vi "Get File Path.vi"(8 "error in (no error)":errorcluster, 11 "DSF Configuration Reference in":T1) -> (0 "error out":errorcluster, 2 "file path":path, 3 "DSF Configuration Reference out":T1, 5 "need update":bool)   [LabVIEW 2017, in "DSF Configuration API.lvlib"]
uses:
  DSF Configuration API.lvlib
  Controls/Session/DSF Configuration Reference.ctl
  Controls/DSF File Format/Internal.DSF Configuration.ctl
  Public/Controls/DSF Version Info.ctl
  Controls/DSF File Format/Internal.DSF Plugin with ID.ctl
  Controls/DSF File Format/Internal.DSF Plugin Info.ctl
  Public/Controls/DSF Timing Info.ctl
  Controls/DSF File Format/Internal.DSF Group with ID.ctl
  Controls/DSF File Format/Internal.DSF Group Info.ctl
  Controls/DSF File Format/Internal.DSF Transfer with ID.ctl
  Controls/DSF File Format/Internal.DSF Transfer Info.ctl
  Controls/DSF File Format/Internal.DSF Channel with ID.ctl
  Controls/DSF File Format/Internal.DSF Channel Info.ctl
  Controls/DSF File Format/Internal.DSF Settings with ID.ctl
  Controls/DSF File Format/Internal.DSF Settings Info.ctl
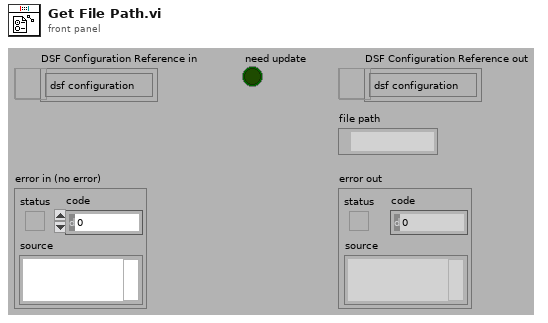
[diagram p1: front panel]
types:
  T1 = typedef "DSF Configuration API.lvlib/DSF Configuration Reference.ctl" = refnum<data-value>
  T2 = typedef "DSF Configuration API.lvlib/Internal.DSF Configuration.ctl" = cluster{"dsfversion":T3, "version":T3, "plugins":T4[], "groups":T7[], "transfers":T9[], "channels":T11[], "settings":T13[]}
  T3 = typedef "DSF Configuration API.lvlib/DSF Version Info.ctl" = cluster{"major":u32, "minor":u32, "fix":u32, "build":string}
  T4 = typedef "DSF Configuration API.lvlib/Internal.DSF Plugin with ID.ctl" = cluster{"id":string, "values":T5}
  T5 = typedef "DSF Configuration API.lvlib/Internal.DSF Plugin Info.ctl" = cluster{"type":string, "timing":T6, "group ids":string[], "settings id":string}
  T6 = typedef "DSF Configuration API.lvlib/DSF Timing Info.ctl" = cluster{"priority":u64, "decimation":u64, "offset":u64}
  T7 = typedef "DSF Configuration API.lvlib/Internal.DSF Group with ID.ctl" = cluster{"id":string, "values":T8}
  T8 = typedef "DSF Configuration API.lvlib/Internal.DSF Group Info.ctl" = cluster{"direction":i32, "timing":T6, "transfer ids":string[], "settings id":string}
  T9 = typedef "DSF Configuration API.lvlib/Internal.DSF Transfer with ID.ctl" = cluster{"id":string, "values":T10}
  T10 = typedef "DSF Configuration API.lvlib/Internal.DSF Transfer Info.ctl" = cluster{"byte order":i32, "channel ids":string[], "settings id":string}
  T11 = typedef "DSF Configuration API.lvlib/Internal.DSF Channel with ID.ctl" = cluster{"id":string, "values":T12}
  T12 = typedef "DSF Configuration API.lvlib/Internal.DSF Channel Info.ctl" = cluster{"count":u64, "buffer offset":u64, "data type":i32, "settings id":string}
  T13 = typedef "DSF Configuration API.lvlib/Internal.DSF Settings with ID.ctl" = cluster{"id":string, "values":T14}
  T14 = typedef "DSF Configuration API.lvlib/Internal.DSF Settings Info.ctl" = cluster{"key":string, "value":string}[]
  T15 = cluster{"dsf configuration":T2, "path":path, "dirty":bool}
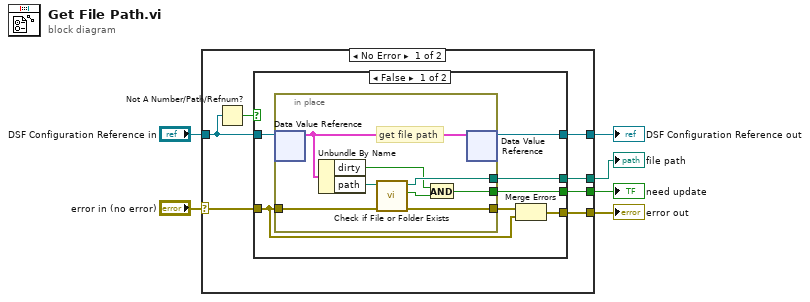
[diagram p0: block diagram]
diagram:
  n1 = case shown="No Error" "error in (no error)" {
    selector: "error in (no error)" -> [w10 w31]
    tunnel: "DSF Configuration Reference in" -> [w8 w32]
    tunnel: [w13 _] -> w6
    tunnel: [w11 w32] -> w2
    tunnel: [w12 w31] -> w4
    tunnel: [w9 _] -> w1
    frame No Error {
      n2 = Not A Number/Path/Refnum?(number/path/refnum=w8) -> (NaN/Path/Refnum?=w7:bool)
      n3 = case shown="False" w7 {
        tunnel: [w19 _] -> w13
        tunnel: [w16 w29] -> w12
        tunnel: w8 -> [w15 w30]
        tunnel: [w14 w30] -> w11
        tunnel: w10 -> [w20 w29]
        tunnel: [w18 _] -> w9
        frame False {
          n4 = in-place {
            in-place-border: w20 -> [w28]
            in-place-border: [w26] -> w19
            in-place-border: [w25] -> w18
            in-place-border: [w22] -> w17
            # "get file path"
            n5 = in-place-dvr #1(w15) -> (w21:T15)  [unwired: 1 out]
            n6 = Unbundle By Name(w21) -> ("dirty"=w24:bool, "path"=w27:path)
            n7 = call <vilib>:"Check if File or Folder Exists.vi"("error in (no error)"=w28, "path"=w27) -> ("error out"=w22:errorcluster, "file or folder exists?"=w23:bool, "dup path"=w26:path)  [unwired: 7 out]
            n8 = And(x=w24, y=w23) -> (x .and. y?=w25:bool)
            n9 = in-place-dvr #1(w21) -> (w14:T1)  [unwired: 1 out]
          }
          n10 = Merge Errors(w17, w20) -> (w16:errorcluster)
        }
        frame True {
        }
      }
    }
    frame Error {
    }
  }
  "error out" <- w4
  "file path" <- w6
  "DSF Configuration Reference out" <- w2
  "need update" <- w1
